vi "Fluke Multimeter Check Status (No Objects).vi"(8 "error in (no error)":errorcluster, 11 "input cluster":T1) -> (0 "error out":errorcluster, 1 "Status":string, 2 "Ready?":bool, 3 "output cluster":T1)   [LabVIEW 2009]
doc: "(Dynamic) Check if the instrument is powered on and update its member data with the instrument's current status. Optionally return a text status message."
uses:
  Global/GPIB Numbers.vi
  Fluke 8840/Fluke 8840.lvlib
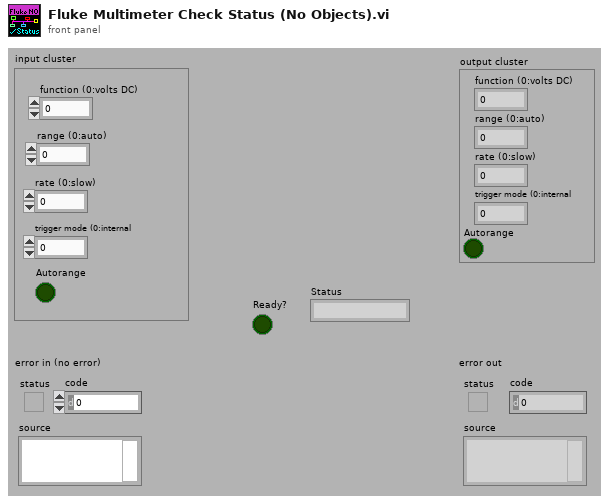
[diagram p1: front panel]
types:
  T1 = cluster{"function (0:volts DC)":i16, "range (0:auto)":i16, "rate (0:slow)":i16, "trigger mode (0:internal":i16, "Autorange":bool}
  T2 = typedef "GPIB Type Def.ctl" = cluster{"Name":string, "bus":dbl, "GPIB":dbl, "GPIB as string":string, "byte":i32, "VISA Resource Name":refnum<visa-resource-name>}
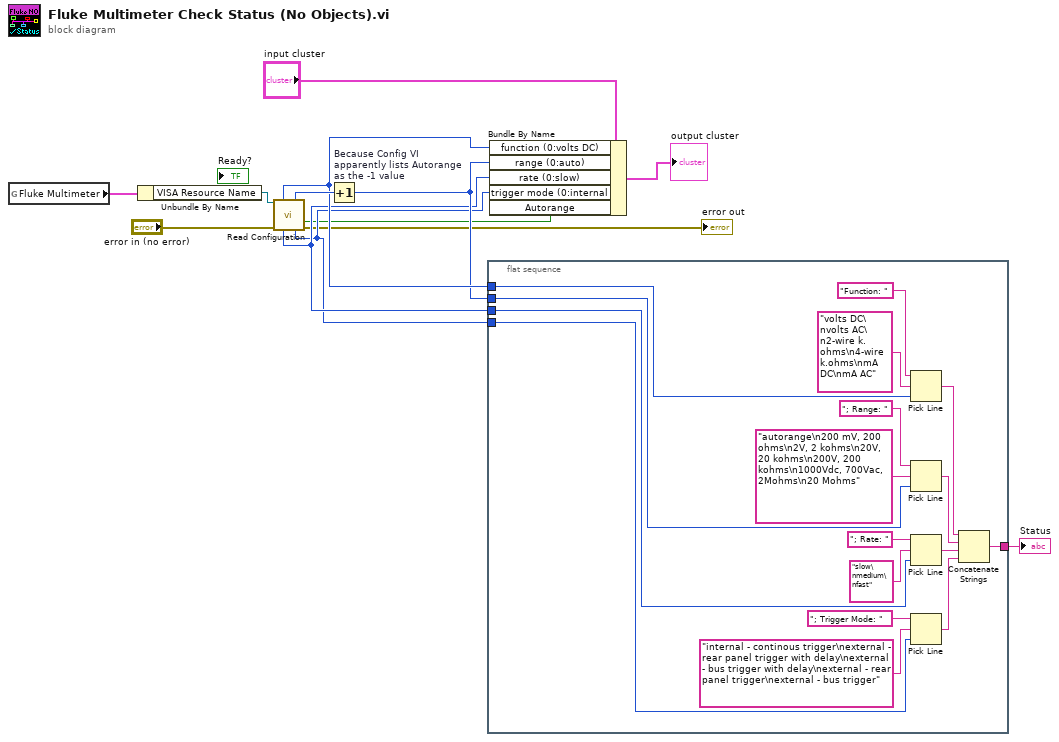
[diagram p0: block diagram]
diagram:
  n1 = global read "GPIB Numbers.vi" "Fluke Multimeter"() -> (w2:T2)
  n2 = Unbundle By Name(w2) -> ("VISA Resource Name"=w1:refnum<visa-resource-name>)
  n3 = call "Read Configuration.vi"("VISA resource name"=w1, "error in (no error)"="error in (no error)") -> ("function"=w11:i32, "range"=w12:i32, "autorange"=w7:bool, "rate"=w9:i32, "trigger mode"=w8:i32, "error out"=→"error out":errorcluster)  [unwired: 8 out]
  n4 = Increment "Because Config VI\napparently lists Autorange\nas the -1 value"(x=w12) -> (x+1=w10:i32)
  n5 = flat-sequence {
    tunnel: [w28] -> w13
    tunnel: w11 -> [w26]
    tunnel: w10 -> [w23]
    tunnel: w9 -> [w18]
    tunnel: w8 -> [w17]
    frame #0 {
      n6 = Pick Line(string ("")="Function: ", multi-line string="volts DC\nvolts AC\n2-wire k.ohms\n4-wire k.ohms\nmA DC\nmA AC", line index=w26) -> (output string=w29:string)
      n7 = Pick Line(string ("")="; Range: ", multi-line string="autorange\n200 mV, 200 ohms\n2V, 2 kohms\n20V, 20 kohms\n200V, 200 kohms\n1000Vdc, 700Vac, 2Mohms\n20 Mohms", line index=w23) -> (output string=w22:string)
      n8 = Pick Line(string ("")="; Rate: ", multi-line string="slow\nmedium\nfast", line index=w18) -> (output string=w15:string)
      n9 = Pick Line(string ("")="; Trigger Mode: ", multi-line string="internal - continous trigger\nexternal - rear panel trigger with delay\nexternal - bus trigger with delay\nexternal - rear panel trigger\nexternal - bus trigger", line index=w17) -> (output string=w14:string)
      n10 = Concatenate Strings(w29, w22, w15, w14) -> (w28:string)
    }
  }
  n11 = Bundle By Name(cluster="input cluster", "function (0:volts DC)"=w11, "range (0:auto)"=w10, "rate (0:slow)"=w9, "trigger mode (0:internal"=w8, "Autorange"=w7) -> (→"output cluster":T1)
  "Status" <- w13
